vi "Remove_FF_lone_spikes.vi"(3 "ADC Frequency Hz":dbl=1000.0 format="%.2f", 4 "Bkgnd variance":dbl format="%.6f", 5 "AIC index":i32, 6 "Time Trace":dbl[](array[numeric])) -> (0 "No Removed":i32, 2 "Filtered Time Trace":dbl[](array[numeric]))   [LabVIEW 2014]
uses:
  Globals/Meas_global.vi
panel:
  out "Time Trace":dbl[][](graph)
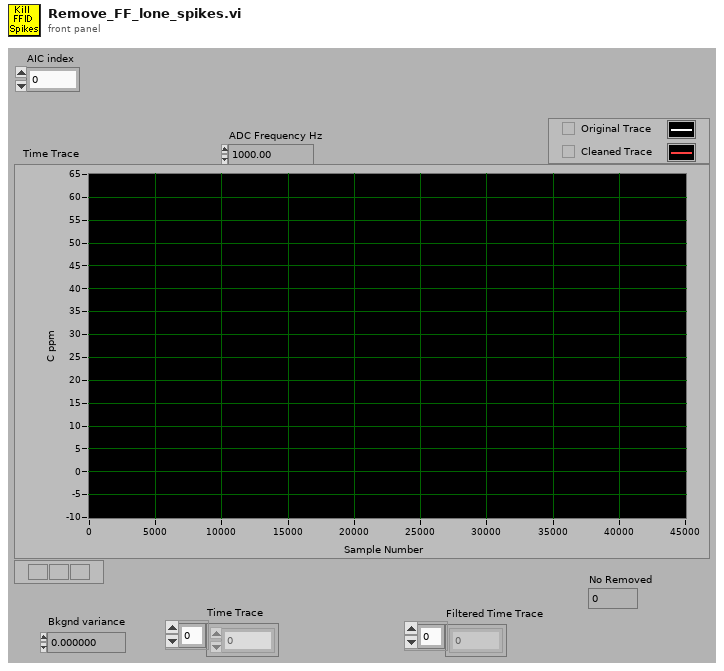
[diagram p1: front panel]
types:
  T1 = typedef "Analysis_info_cluster.ctl" = cluster{"Colour":u32, "Inst type":T2, "Inst name":string, "Symbol":string, "Code name":string, "Extra Info":string, "Inst Array":T3, "Extra Titles":string[], "Extra Values":string[], "U":dbl, "u^2":dbl, "u^3":dbl, "u^4":dbl, "Skew_u":dbl, "Kurt_u":dbl, "Sd Error in Mean":dbl, "% u'/U":dbl, "X":dbl, "Y":dbl, "Z":dbl, "Timescale integral to 25%":dbl, "Sd Error in Variance":dbl, "Calib File":path, "Calib Constants":dbl[], "Output Position":bool, "Full Stats":bool, "Av Sampling Rate":dbl, "Av No of Samples":dbl, "Total Meas Time (s)":dbl, "ADAM Ch Name":string}
  T2 = typedef "Inst_type.ctl" = enum16{"Propeller anemometer", "Raw voltage", "Pressure Transducer", "Pitot-static tube", "Preston tube", "Hot wire", "Cross wire 1", "Cross wire 2", "Generic Linear", "Generic Polynomial", "Generic BackPoly", "Fast FID", "Thermocouple", "Cold wire", "Pulsed Wire", "LDA Vel", "LDA Tran time", "LDA Arr time"}
  T3 = typedef "Instrument_Array.ctl" = enum16{"PWA", "LDA", "Analogue"}
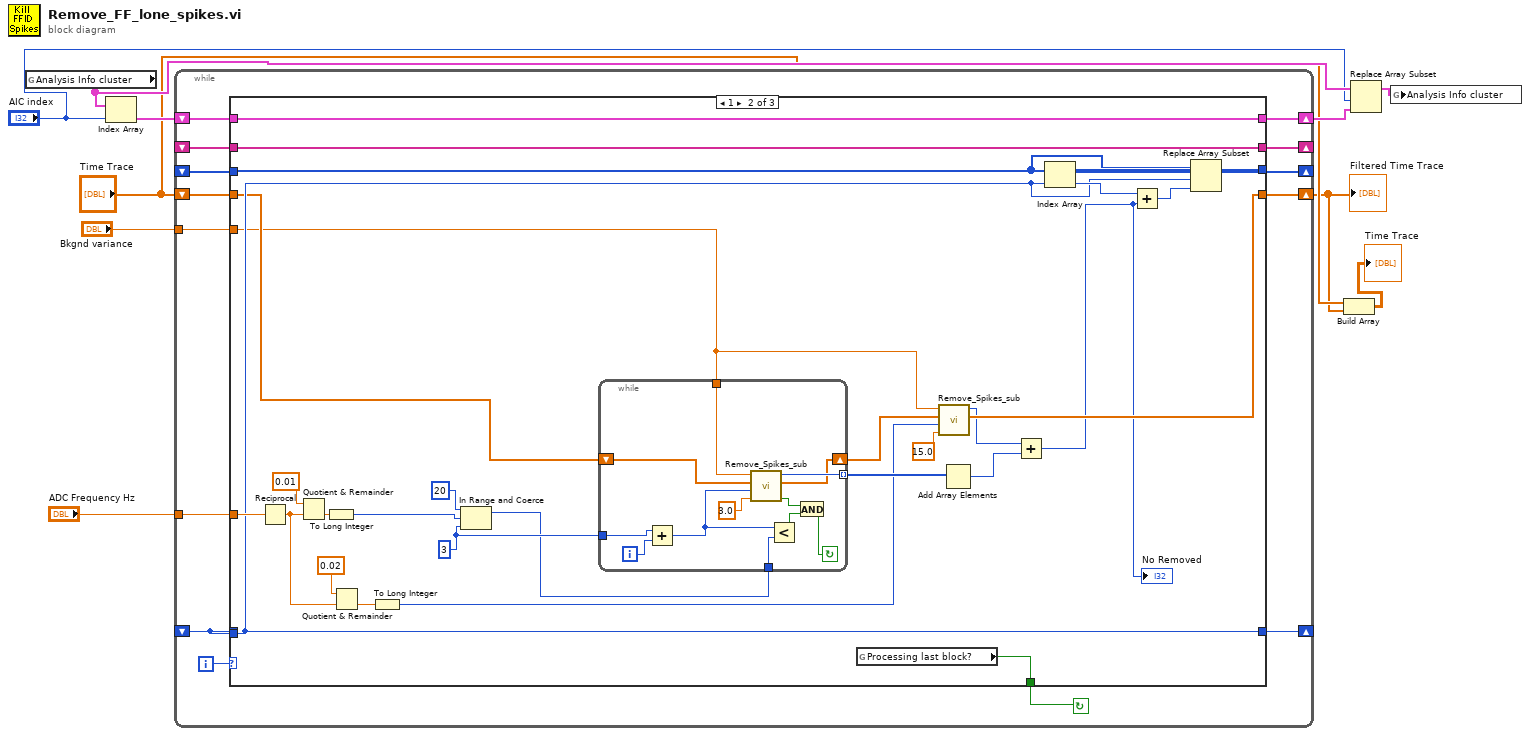
[diagram p0: block diagram]
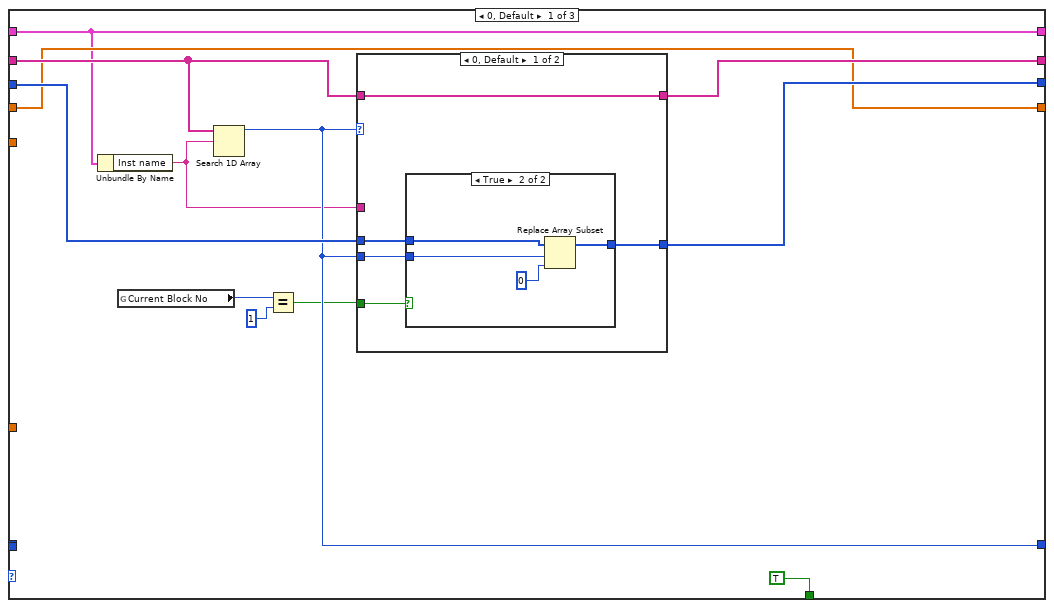
[diagram p2: hidden frame]
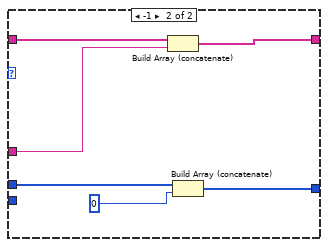
[diagram p4: hidden frame]
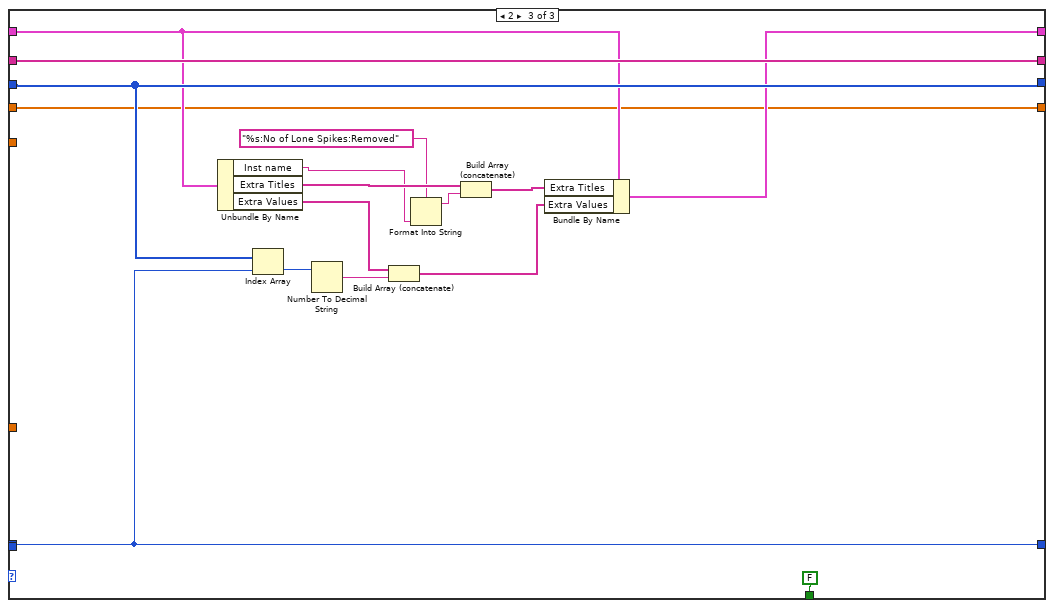
[diagram p5: hidden frame]
diagram:
  n1 = global read "Meas_global.vi" "Analysis Info cluster"() -> (w7:T1[])
  n2 = Index Array(array=w7, index="AIC index") -> (element=w8:T1)
  n3 = while {
    shift-left: _ -> [w21]
    shift-right: [w23] -> _
    shift-right: [w19] -> _
    shift-left: _ -> [w20]
    shift-right: [w17] -> _
    shift-left: _ -> [w18]
    shift-right: [w15] -> w6
    shift-left: w8 -> [w16]
    tunnel: "Bkgnd variance" -> [w14]
    shift-right: [w12] -> w2
    shift-left: "Time Trace" -> [w13]
    tunnel: "ADC Frequency Hz" -> [w11]
    i -> [w24]
    stop <- w22 continue-if-true
    n4 = case shown="1" w24 {
      tunnel: [w29 w71 w106] -> w23
      tunnel: [TRUE w70 FALSE ("Processing last block?")] -> w22
      tunnel: w21 -> [_ _ w106]
      tunnel: w21 -> [_ w71 _]
      tunnel: w20 -> [w33 w80 w104]
      tunnel: [w32 w80 w104] -> w19
      tunnel: w18 -> [w31 w79 w103]
      tunnel: [w30 w77 w103] -> w17
      tunnel: w16 -> [w26 w76 w100]
      tunnel: [w26 w76 w102] -> w15
      tunnel: w14 -> [_ w63 _]
      tunnel: w13 -> [w27 w67 w96]
      tunnel: [w27 w56 w96] -> w12
      tunnel: w11 -> [_ w74 _]
      frame 0, Default {
        n5 = Unbundle By Name(w26) -> ("Inst name"=w25:string)
        n6 = global read "Meas_global.vi" "Current Block No"() -> (w35:i32)
        n7 = Search 1D Array(1D array=w33, element=w25) -> (index of element=w29:i32)  [unwired: 1 out]
        n8 = Equal?(x=w35, y=1) -> (x = y?=w28:bool)
        n9 = case shown="0, Default" w29 {
          tunnel: w33 -> [w41 w52]
          tunnel: w25 -> [_ w51]
          tunnel: [w41 w50] -> w32
          tunnel: w31 -> [w40 w49]
          tunnel: [w39 w48] -> w30
          tunnel: w29 -> [w38 _]
          tunnel: w28 -> [w37 _]
          frame 0, Default {
            n10 = case shown="True" w37 {
              tunnel: w40 -> [w42 w46]
              tunnel: [w42 w45] -> w39
              tunnel: w38 -> [_ w44]
              frame False {
              }
              frame True {
                n11 = Replace Array Subset(array=w46, new element=0, index=w44) -> (w45:i32[])
              }
            }
          }
          frame -1 {
            n12 = Build Array (concatenate)(w52, w51) -> (w50:string[])
            n13 = Build Array (concatenate)(w49, 0) -> (w48:i32[])
          }
        }
      }
      frame 1 {
        w65 = 3 ("lower limit")
        n14 = Reciprocal(x=w74) -> (1/x=w59:dbl)
        n15 = Quotient & Remainder(x=0.01, y=w59) -> (floor(x/y)=w72:dbl)  [unwired: 1 out]
        n16 = To Long Integer(number=w72) -> (32bit integer=w68:i32)
        n17 = Quotient & Remainder(x=0.02, y=w59) -> (floor(x/y)=w58:dbl)  [unwired: 1 out]
        n18 = To Long Integer(number=w58) -> (32bit integer=w57:i32)
        n19 = In Range and Coerce(upper limit=20, x=w68, lower limit=w65) -> (coerced(x)=w64:i32)  [unwired: 1 out]
        n20 = while {
          tunnel: [w92] -> w66 mode=indexing
          shift-right: [w91] -> w62
          shift-left: w67 -> [w86]
          tunnel: w65 -> [w89]
          tunnel: w64 -> [w87]
          tunnel: w63 -> [w82]
          i -> [w90]
          stop <- w83 continue-if-true
          n21 = Add(x=w89, y=w90) -> (x+y=w88:i32)
          n22 = call "Remove_Spikes_sub.vi"("Number of Sigma to cut after"=3.0, "Number of samples"=w88, "Time Trace in"=w86, "Bkgnd Variance"=w82) -> ("Checked"=w85:bool, "Time Trace out"=w91:dbl[], "Numeric out"=w92:i32)  [unwired: 5 in]
          n23 = Less?(x=w88, y=w87) -> (x < y?=w84:bool)
          n24 = And(x=w85, y=w84) -> (x .and. y?=w83:bool)
        }
        n25 = global read "Meas_global.vi" "Processing last block?"() -> (w70:bool)
        n26 = call "Remove_Spikes_sub.vi"("Number of Sigma to cut after"=15.0, "Number of samples"=w57, "Time Trace in"=w62, "Bkgnd Variance"=w63) -> ("Time Trace out"=w56:dbl[], "Numeric out"=w55:i32)  [unwired: 5 in, 1 out]
        n27 = Add Array Elements(numeric array=w66) -> (sum=w54:i32)
        n28 = Add(x=w55, y=w54) -> (x+y=w53:i32)
        "No Removed" <- w53
        n29 = Index Array(array=w79, index=w71) -> (element=w78:i32)
        n30 = Add(x=w78, y=w53) -> (x+y=w75:i32)
        n31 = Replace Array Subset(array=w79, new element=w75, index=w71) -> (w77:i32[])
      }
      frame 2 {
        n32 = Unbundle By Name(w100) -> ("Inst name"=w94:string, "Extra Titles"=w99:string[], "Extra Values"=w98:string[])
        n33 = Index Array(array=w103, index=w106) -> (element=w105:i32)
        n34 = Number To Decimal String(number=w105) -> (decimal integer string=w107:string)  [unwired: 1 out]
        n35 = Build Array (concatenate)(w98, w107) -> (w97:string[])
        n36 = Format Into String(format string="%s:No of Lone Spikes:Removed", w94) -> (resulting string=w95:string)  [unwired: 2 in, 1 out]
        n37 = Build Array (concatenate)(w99, w95) -> (w101:string[])
        n38 = Bundle By Name(cluster=w100, "Extra Titles"=w101, "Extra Values"=w97) -> (w102:T1)
      }
    }
  }
  "Filtered Time Trace" <- w2
  n39 = Build Array("Time Trace", w2) -> (→"Time Trace":dbl[][])
  n40 = Replace Array Subset(array=w7, new element=w6, index="AIC index") -> (w4:T1[])
  n41 = global write "Meas_global.vi" "Analysis Info cluster"(w4) -> ()
